vi "CreateUserEventMessage.vi"(8 "error in":errorcluster, 9 "initial message data []":variant[](array[variant]), 10 "initial message names []":string[](array[string])) -> (0 "error out":errorcluster, 3 "message ref out":refnum<class "CLM_LocalMessage_UserEvent.lvclass">)   [LabVIEW 2013, in "CLM_LocalMessage_UserEvent.lvclass"]
uses:
  CLM_LocalMessage_UserEvent.lvclass
  LocalMessage/Message.ctl
  CLM_LocalMessage_UserEvent.lvclass/CLM_LocalMessage_UserEvent.ctl
  SendUserEventMessage.vi
  LocalMessage/BundleMessageCluster.vi
  SendUserEventMessage_Cluster.vi
  LocalMessage/CLM_LocalMessage.lvclass
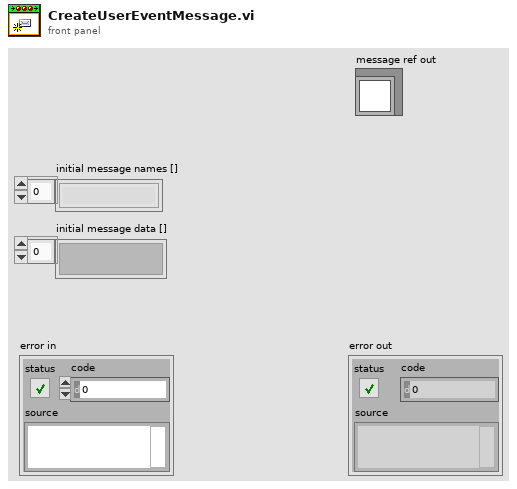
[diagram p1: front panel]
types:
  T1 = typedef "CLM_LocalMessage.lvclass/Message.ctl" = cluster{"name":string, "data":variant, "attributes":variant, "urgent":bool}
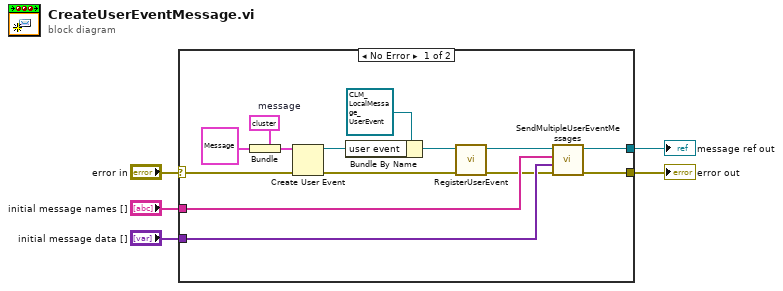
[diagram p0: block diagram]
diagram:
  n1 = case shown="No Error" "error in" {
    selector: "error in" -> [w16 w20]
    tunnel: "initial message names []" -> [w19 _]
    tunnel: "initial message data []" -> [w18 _]
    tunnel: [w17 w20] -> w2
    tunnel: [w10 _] -> w1
    frame No Error {
      w13 = cluster{"message":T1} {"message"={"name"="", "data"=variant, "attributes"=variant, "urgent"=FALSE}}  # message
      n2 = Bundle(cluster=w13, "message"=T1 {"name"="", "data"=variant, "attributes"=variant, "urgent"=FALSE}) -> (w14:cluster{"message":T1})
      n3 = Create User Event(user event datatype=w14, error in=w16) -> (user event=w11:refnum<user-event>, error out=w7:errorcluster)
      n4 = Bundle By Name(cluster=refnum<class "CLM_LocalMessage_UserEvent.lvclass"> refnum ("message user event out"), "user event"=w11) -> (w9:refnum<class "CLM_LocalMessage_UserEvent.lvclass">)
      n5 = call "RegisterUserEvent.vi"("error in"=w7, "message ref in"=w9) -> ("error out"=w6:errorcluster, "message ref out"=w8:refnum<class "CLM_LocalMessage_UserEvent.lvclass">)  [unwired: 8 in]
      n6 = call "SendMultipleUserEventMessages.vi"("error in"=w6, "message data []"=w18, "message names []"=w19, "message ref in"=w8) -> ("error out"=w17:errorcluster, "message ref out"=w10:refnum<class "CLM_LocalMessage_UserEvent.lvclass">)  [unwired: 6 in]
    }
    frame Error {
    }
  }
  "error out" <- w2
  "message ref out" <- w1
